vi "Fit Spline to Velocity Profile.vi"(8 "time":dbl[](array[numeric]), 9 "vel positions":sgl[](array[numeric]), 10 "s(t)":dbl[](array[numeric]), 11 "t flat":sgl[](array[numeric])) -> (2 "time unflat":cluster{dbl[]}[](array[cluster]), 3 "y unflat":cluster{dbl[]}[](array[cluster]))   [LabVIEW 2025]
panel:
  in  "debug?":bool
  in  "poly degree":i32=50
  out "Points":cluster{"s(t)":dbl[], "t flat":sgl[]}(graph)
  out "Fitted":cluster{"vel positions":sgl[], "y":dbl[]}(graph)
  out "y":dbl[](array[numeric])
  # "max polynomial degree"
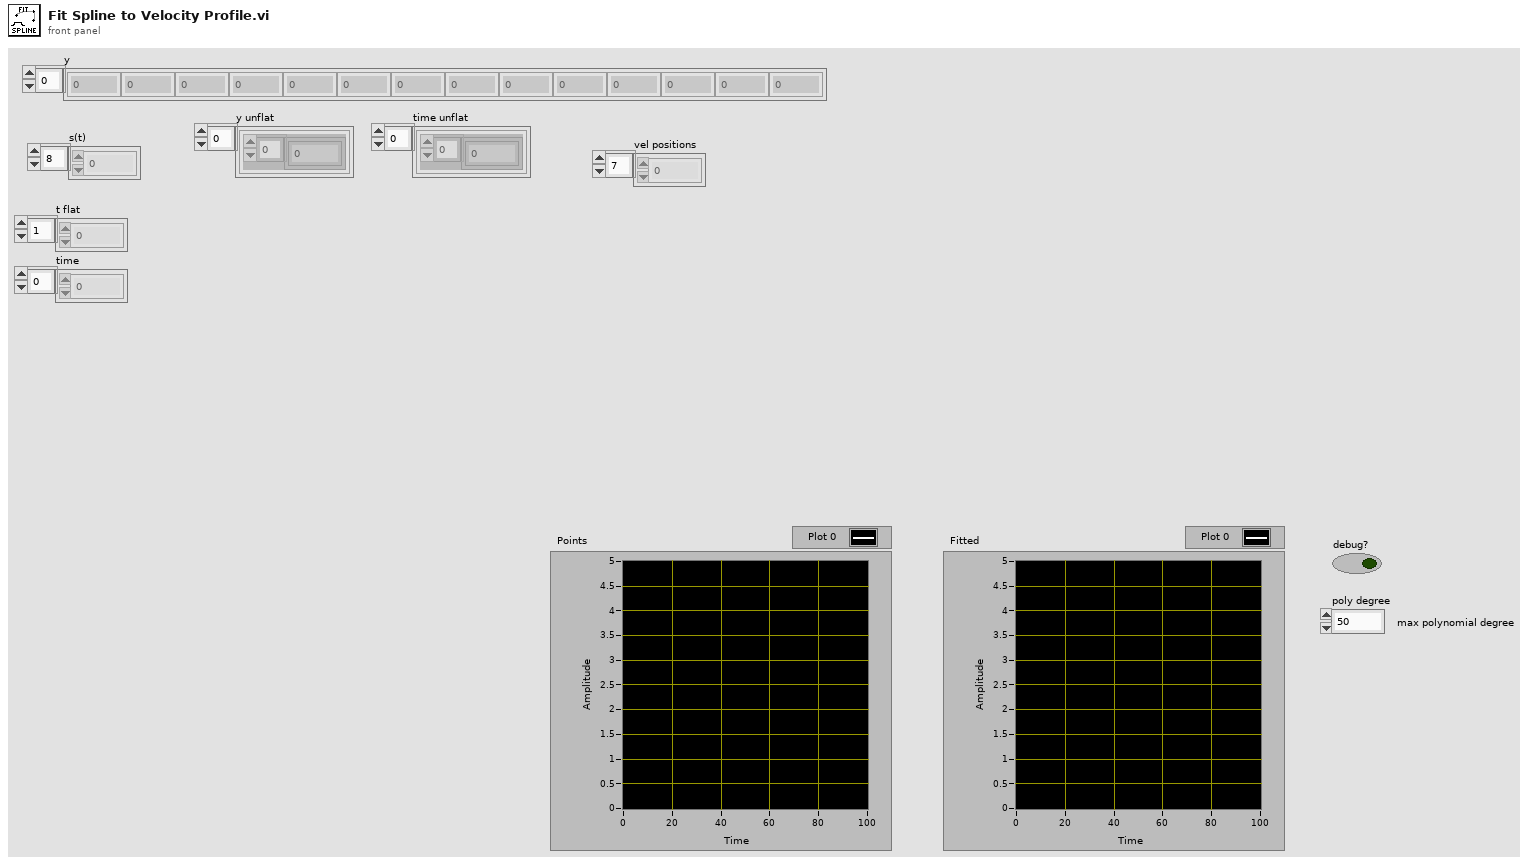
[diagram p1: front panel]
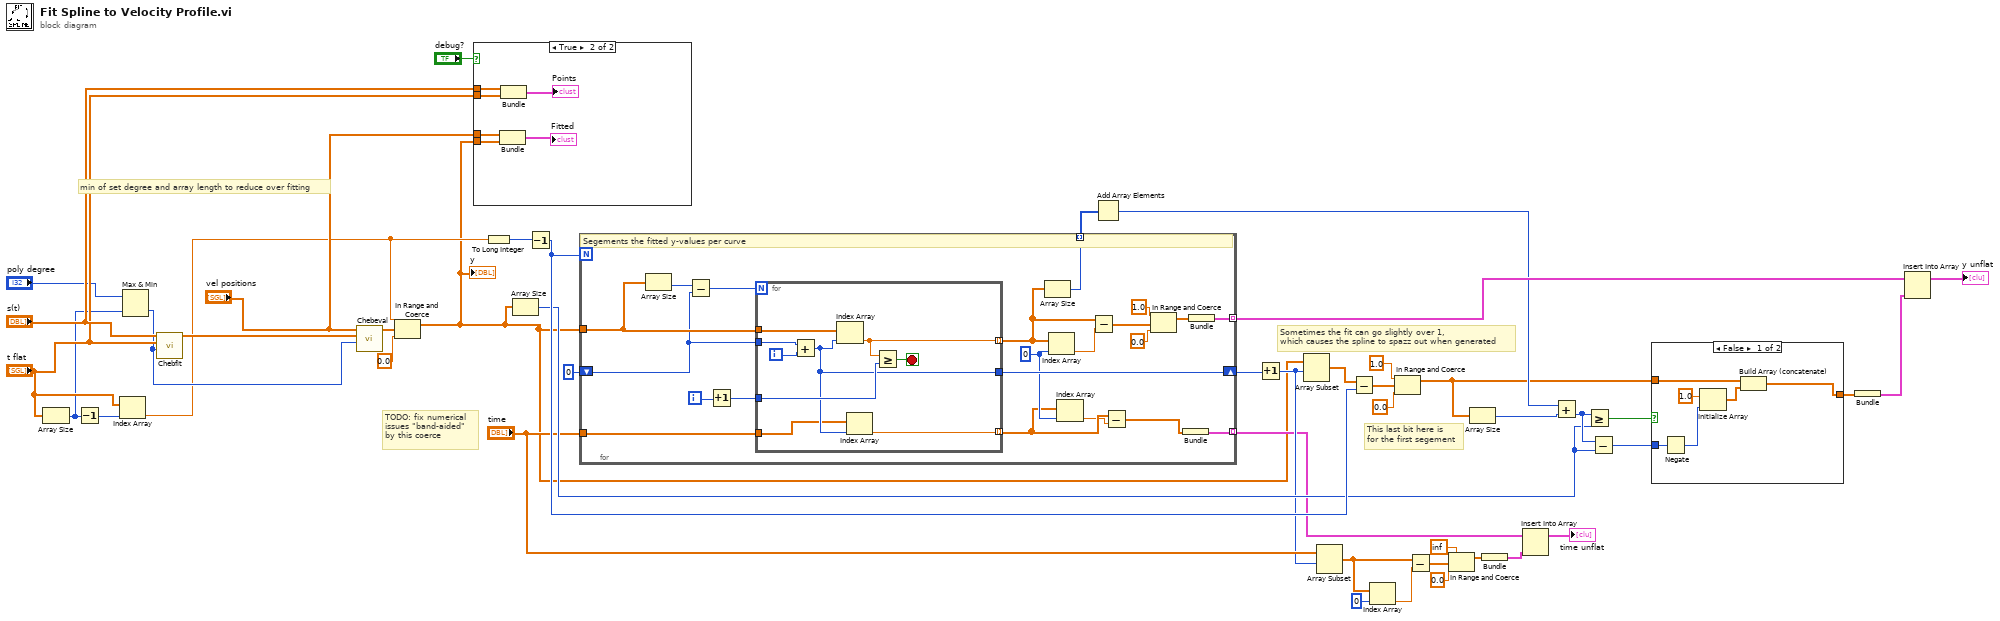
[diagram p0: block diagram]
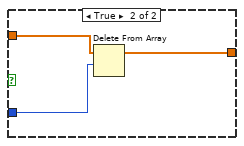
[diagram p3: hidden frame]
diagram:
  # "TODO: fix numerical \nissues \"band-aided\"\nby this coerce"
  # "min of set degree and array length to reduce over fitting"
  # "This last bit here is\nfor the first segement"
  # "Sometimes the fit can go slightly over 1,\nwhich causes the spline to spazz out when generated"
  n1 = Array Size(array="t flat") -> (size(s)=w7:i32)
  n2 = Decrement(x=w7) -> (x-1=w43:i32)
  n3 = Index Array(array="t flat", index=w43) -> (element=w4:sgl)
  n4 = Max & Min(x="poly degree", y=w7) -> (min(x,y)=w6:i32)  [unwired: 1 out]
  n5 = call "Chebfit.vi"("degree"=w6, "Y"="t flat", "X"="s(t)") -> ("C"=w24:dbl[])  [unwired: 8 in]
  n6 = call "Chebeval.vi"("degree"=w6, "Cheby weights"=w24, "x"="vel positions") -> ("y"=w5:dbl[])  [unwired: 8 in]
  n7 = In Range and Coerce(upper limit=w4, x=w5, lower limit=sgl 0.0 ("element")) -> (coerced(x)=w2:dbl[])  [unwired: 1 out]
  "y" <- w2
  n8 = case shown="True" "debug?" {
    tunnel: "vel positions" -> [_ w51]
    tunnel: "s(t)" -> [_ w50]
    tunnel: "t flat" -> [_ w49]
    tunnel: w2 -> [_ w48]
    frame False {
    }
    frame True {
      n9 = Bundle("vel positions"=w51, w48) -> (→"Fitted":cluster{"vel positions":sgl[], dbl[]})  [unwired: 1 in]
      n10 = Bundle("s(t)"=w50, "t flat"=w49) -> (→"Points":cluster{"s(t)":dbl[], "t flat":sgl[]})  [unwired: 1 in]
    }
  }
  n11 = To Long Integer(number=w4) -> (32bit integer=w42:i32)
  n12 = Array Size(array=w2) -> (size(s)=w28:i32)
  n13 = Decrement(x=w42) -> (x-1=w37:i32)
  n14 = for {
    N: w37 -> [_]
    tunnel: w2 -> [w72]
    shift-right: [w68] -> w40
    shift-left: 0 -> [w69]
    tunnel: [w62] -> w41 mode=indexing
    tunnel: [w60] -> w44 mode=indexing
    tunnel: "time" -> [w57]
    tunnel: [w56] -> w14 mode=indexing
    i -> [w59]
    w55 = 0 ("index")
    # "Segements the fitted y-values per curve"
    n15 = Array Size(array=w72) -> (size(s)=w71:i32)
    n16 = Subtract(x=w71, y=w69) -> (x-y=w70:i32)
    n17 = Increment(x=w59) -> (x+1=w58:i32)
    n18 = for {
      N: w70 -> [_]
      tunnel: w72 -> [w79]
      tunnel: w69 -> [w80]
      tunnel: w58 -> [w78]
      tunnel: [w75] -> w68
      tunnel: [w76] -> w61 mode=indexing
      tunnel: w57 -> [w74]
      tunnel: [w73] -> w54 mode=indexing
      i -> [w81]
      stop <- w77 stop-if-true
      n19 = Add(x=w80, y=w81) -> (x+y=w75:i32)
      n20 = Index Array(array=w79, index=w75) -> (element=w76:dbl)
      n21 = Index Array(array=w74, index=w75) -> (element=w73:dbl)
      n22 = Greater Or Equal?(x=w76, y=w78) -> (x >= y?=w77:bool)
    }
    n23 = Array Size(array=w61) -> (size(s)=w60:i32)
    n24 = Index Array(array=w61, index=w55) -> (element=w67:dbl)
    n25 = Index Array(array=w54, index=w55) -> (element=w53:dbl)
    n26 = Subtract(x=w61, y=w67) -> (x-y=w66:dbl[])
    n27 = Subtract(x=w54, y=w53) -> (x-y=w52:dbl[])
    n28 = In Range and Coerce(upper limit=1.0, x=w66, lower limit=0.0) -> (coerced(x)=w63:dbl[])  [unwired: 1 out]
    n29 = Bundle(w52) -> (w56:cluster{dbl[]})  [unwired: 1 in]
    n30 = Bundle(w63) -> (w62:cluster{dbl[]})  [unwired: 1 in]
  }
  n31 = Add Array Elements(numeric array=w44) -> (sum=w32:i32)
  n32 = Increment(x=w40) -> (x+1=w21:i32)
  n33 = Array Subset(array=w2, index=w21) -> (w38:dbl[])  [unwired: 1 in]
  n34 = Array Subset(array="time", index=w21) -> (w20:dbl[])  [unwired: 1 in]
  n35 = Subtract(x=w38, y=w37) -> (x-y=w36:dbl[])
  n36 = Index Array(array=w20, index=0) -> (element=w18:dbl)
  n37 = In Range and Coerce(upper limit=1.0, x=w36, lower limit=0.0) -> (coerced(x)=w30:dbl[])  [unwired: 1 out]
  n38 = Subtract(x=w20, y=w18) -> (x-y=w17:dbl[])
  n39 = In Range and Coerce(upper limit=inf, x=w17, lower limit=0.0) -> (coerced(x)=w13:dbl[])  [unwired: 1 out]
  n40 = Array Size(array=w30) -> (size(s)=w33:i32)
  n41 = Bundle(w13) -> (w12:cluster{dbl[]})  [unwired: 1 in]
  n42 = Insert Into Array(array=w14, new element=w12) -> (→"time unflat":cluster{dbl[]}[])  [unwired: 1 in]
  n43 = Add(x=w32, y=w33) -> (x+y=w29:i32)
  n44 = Greater Or Equal?(x=w29, y=w28) -> (x >= y?=w31:bool)
  n45 = Subtract(x=w29, y=w28) -> (x-y=w27:i32)
  n46 = case shown="False" w31 {
    tunnel: w30 -> [w87 w90]
    tunnel: w27 -> [w86 w89]
    tunnel: [w82 w88] -> w25
    frame False {
      n47 = Negate(x=w86) -> (-x=w85:i32)
      n48 = Initialize Array(1.0 ("element"), w85) -> (w83:dbl[])
      n49 = Build Array (concatenate)(w87, w83) -> (w82:dbl[])
    }
    frame True {
      n50 = Delete From Array(array=w90, length=w89) -> (array with subset deleted=w88:dbl[])  [unwired: 1 in, 1 out]
    }
  }
  n51 = Bundle(w25) -> (w26:cluster{dbl[]})  [unwired: 1 in]
  n52 = Insert Into Array(array=w41, new element=w26) -> (→"y unflat":cluster{dbl[]}[])  [unwired: 1 in]
